vi "read_db_selected_events.vi"(8 "error in (no error)":errorcluster, 10 "Small?":bool, 11 "Dust Events":i64[](array[numeric])) -> (0 "error out":errorcluster, 1 "ID Experiment Settings":i32[](array[numeric]), 2 "ID Dust Events":i64[](array[numeric]), 3 "Dust Array":T2[](array[typedef]) {"File Location" items=["Unknown"=-1, "Processing"=0, "Storage"=1]; "Estimate Source" items=["Any Source."=-2, "No Shot"=-1, "Basic Labview Estimate"=0, "IDL Estimate From Andrew"=1, "IDL Estimate From Tobin"=2, "Old Metadata"=3]}, 5 "File Locations":T1[](array[typedef]) items=["Unknown"=-1, "Processing"=0, "Storage"=1])   [LabVIEW 2013]
doc: "Given a set of constraints, this program will return a lot of data about each event that matces the constraints."
uses:
  Public API/Query_Dust_Event.ctl
  Controls/Estimate_source.ctl
  Controls/File_location.ctl
  <userlib>/_OpenG.lib/array/array.llb/Empty 1D Array (I64)__ogtk.vi
  <userlib>/_OpenG.lib/array/array.llb/Reverse 2D Array (Variant)__ogtk.vi
  <vilib>/addons/database/_DB Variant To Data/Database Variant To Data.xnode
panel:
  out "SQL Query Syntax":string
  # "Dust Event"
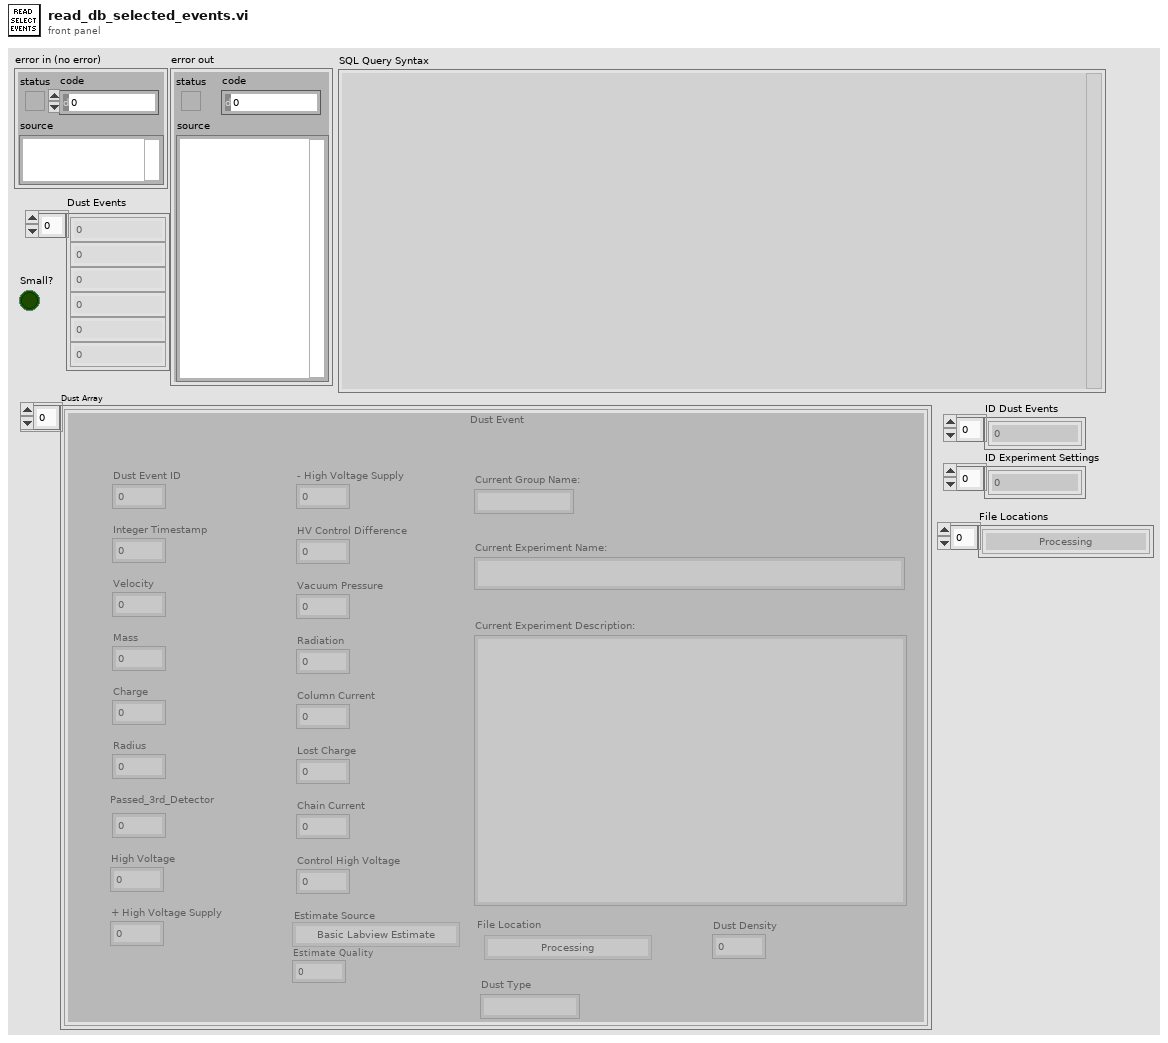
[diagram p1: front panel]
types:
  T1 = typedef "File_location.ctl" = i8
  T2 = typedef "Query_Dust_Event.ctl" = cluster{"Dust Event ID":i64, "Integer Timestamp":i64, "Velocity":sgl, "Mass":sgl, "Charge":sgl, "Radius":sgl, "Passed_3rd_Detector":i8, "High Voltage":sgl, "+ High Voltage Supply":sgl, "- High Voltage Supply":sgl, "HV Control Difference":sgl, "Vacuum Pressure":sgl, "Radiation":sgl, "Column Current":sgl, "Lost Charge":sgl, "Chain Current":sgl, "Control High Voltage":sgl, "Current Group Name:":string, "Current Experiment Name:":string, "Current Experiment Description:":string, "Estimate Source":T3, "Estimate Quality":i8, "File Location":T1, "Dust Type":string, "Dust Density":sgl}
  T3 = typedef "Estimate_source.ctl" = i8
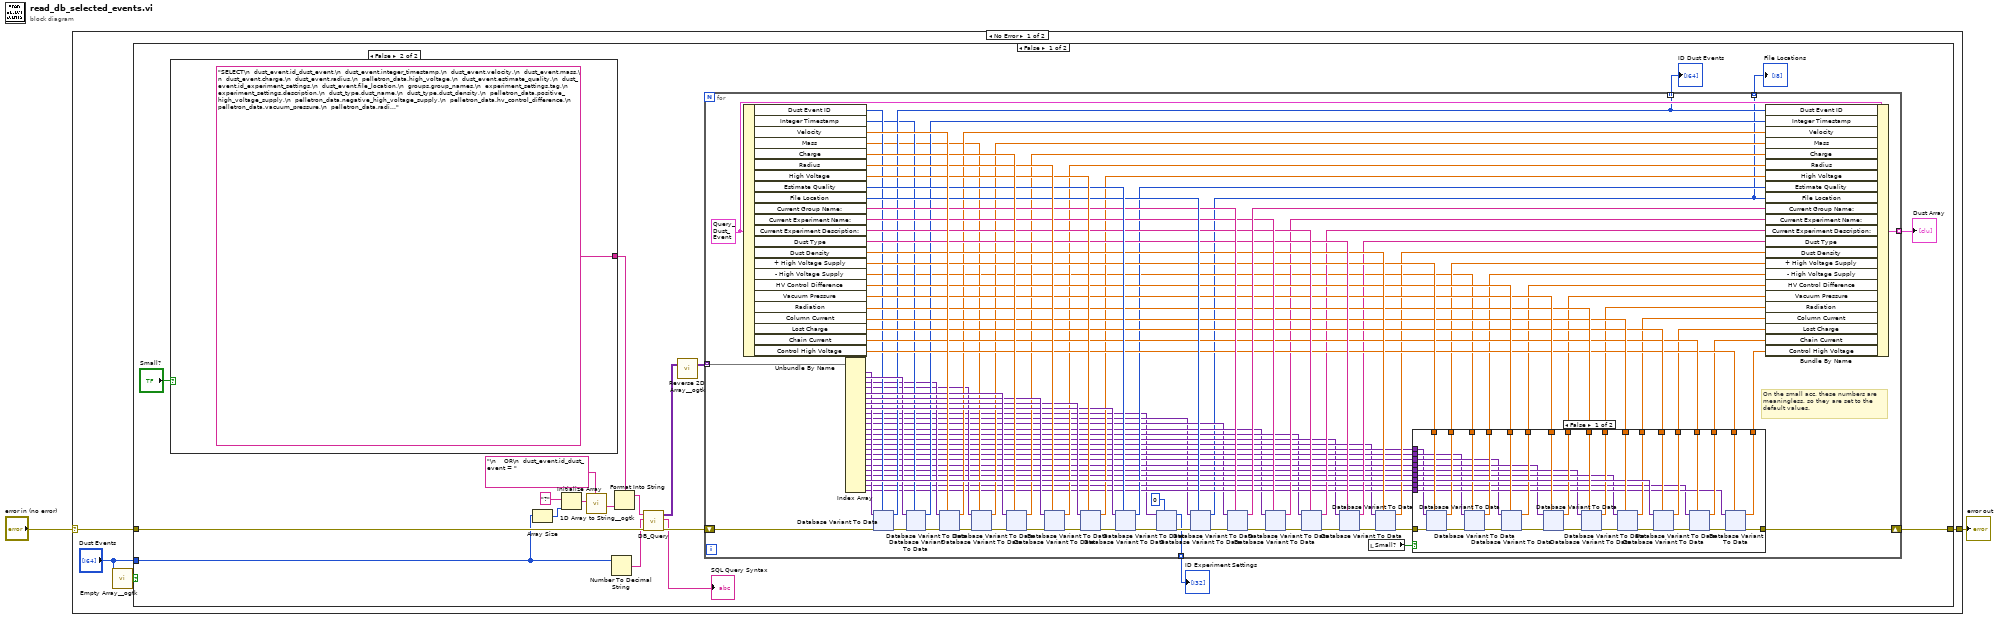
[diagram p0: block diagram]
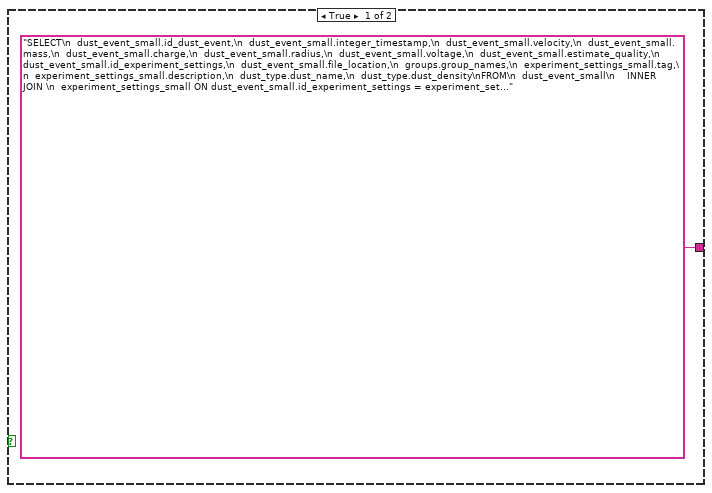
[diagram p3: hidden frame]
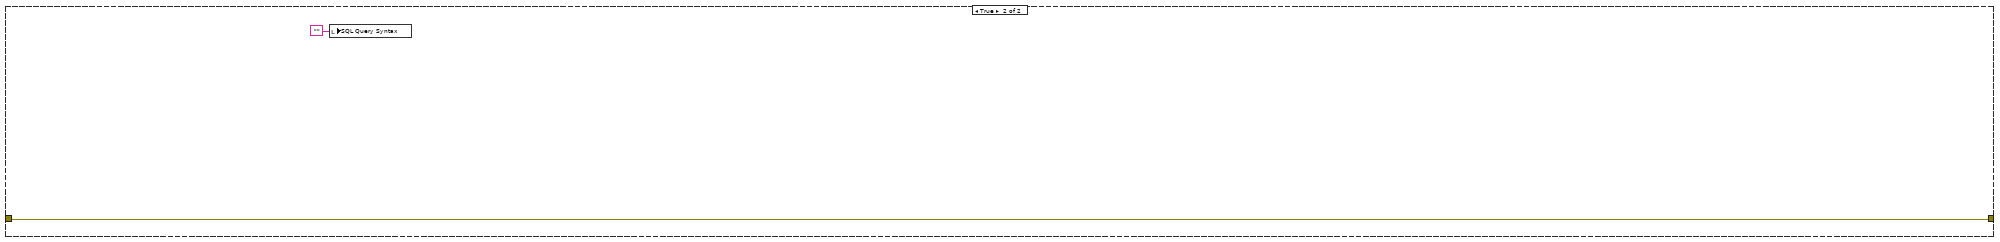
[diagram p4: hidden frame]
diagram:
  n1 = case shown="No Error" "error in (no error)" {
    selector: "error in (no error)" -> [w5 w939]
    tunnel: [w6 w939] -> w1
    frame No Error {
      n2 = call-poly <userlib>:"Empty Array__ogtk.vi"("Array"="Dust Events") -> ("Empty Array?"=w4:bool)  [unwired: 8 in]
      n3 = case shown="False" w4 {
        tunnel: [w24 w938] -> w6
        tunnel: w5 -> [w19 w938]
        tunnel: "Dust Events" -> [w17 _]
        frame False {
          n4 = case shown="False" "Small?" {
            tunnel: ["SELECT\n  dust_event_small.id_dust_event,\n  dust_event_small.integer_timestamp,\n  dust_event_small.velocity,\n  dust_event_small.mass,\n  dust_event_small.charge,\n  dust_event_small.radius,\n  dust_event_small.voltage,\n  dust_event_small.estimate_quality,\n  dust_event_small.id_experiment_settings,\n  dust_event_small.file_location,\n  groups.group_names,\n  experiment_settings_small.tag,\n  experiment_settings_small.description,\n  dust_type.dust_name,\n  dust_type.dust_density\nFROM\n  dust_event_small\n    INNER JOIN \n  experiment_settings_small ON dust_event_small.id_experiment_settings = experiment_settings_small.id_experiment_settings\n    INNER JOIN  \n  groups ON experiment_settings_small.id_groups=groups.id_groups\n    INNER JOIN\n  dust_info_small ON dust_event_small.id_dust_info = dust_info_small.id_dust_info\n  \t\tINNER JOIN\n  dust_type ON dust_info_small.dust_type = dust_type.id_dust_type\nWHERE\n  dust_event_small.id_dust_event = %s; " ("string") "SELECT\n  dust_event.id_dust_event,\n  dust_event.integer_timestamp,\n  dust_event.velocity,\n  dust_event.mass,\n  dust_event.charge,\n  dust_event.radius,\n  pelletron_data.high_voltage,\n  dust_event.estimate_quality,\n  dust_event.id_experiment_settings,\n  dust_event.file_location,\n  groups.group_names,\n  experiment_settings.tag,\n  experiment_settings.description,\n  dust_type.dust_name,\n  dust_type.dust_density,\n  pelletron_data.positive_high_voltage_supply,\n  pelletron_data.negative_high_voltage_supply,\n  pelletron_data.hv_control_difference,\n  pelletron_data.vacuum_pressure,\n  pelletron_data.radiation,\n  pelletron_data.column_current,\n  pelletron_data.lost_charge,\n  pelletron_data.chain_current,\n  pelletron_data.control_high_voltage\nFROM\n  dust_event\n    INNER JOIN \n  experiment_settings ON dust_event.id_experiment_settings = experiment_settings.id_experiment_settings\n    INNER JOIN  \n  groups ON experiment_settings.id_groups=groups.id_groups\n    INNER JOIN\n  pelletron_data ON pelletron_data.id_pelletron_data = dust_event.id_pelletron_data\n    INNER JOIN\n  dust_info ON dust_event.id_dust_info = dust_info.id_dust_info\n\t\t  INNER JOIN\n\t dust_type ON dust_info.dust_type = dust_type.id_dust_type\nWHERE\n  dust_event.id_dust_event = %s; " ("string")] -> w12
            frame True {
            }
            frame False {
            }
          }
          n5 = Array Size(array=w17) -> (size(s)=w15:i32)
          n6 = Initialize Array("?", w15) -> (w14:string[])
          n7 = call <userlib>:"1D Array to String__ogtk.vi"("delimiter (Tab)"="\n    OR\n  dust_event.id_dust_event = ", "Array of Strings"=w14) -> ("delimited string"=w10:string)  [unwired: 9 in]
          n8 = Number To Decimal String(number=w17) -> (decimal integer string=w18:string[])  [unwired: 1 in]
          n9 = Format Into String(format string=w12, w10) -> (resulting string=w11:string)  [unwired: 2 in, 1 out]
          n10 = call "DB_Query.vi"("error in (no error)"=w19, "Parameters"=w18, "Parameterized Query"=w11) -> ("error out"=w22:errorcluster, "Query in Standard Format"=→"SQL Query Syntax":string, "Results"=w21:variant[][])  [unwired: 6 in]
          n11 = call-poly <userlib>:"Reverse 2D Array__ogtk.vi"("Array"=w21) -> ("Reversed Array"=w23:variant[][])  [unwired: 2 in]
          n12 = for {
            tunnel: w23 -> [w119] mode=indexing
            shift-right: [w87] -> w24
            shift-left: w22 -> [w118]
            tunnel: [w92] -> w26 mode=indexing
            tunnel: [w79] -> w9 mode=indexing
            tunnel: [w29] -> w7 mode=indexing
            tunnel: [w28] -> w8 mode=indexing
            w117 = T2 {"Dust Event ID"=0, "Integer Timestamp"=0, "Velocity"=0.0, "Mass"=0.0, "Charge"=0.0, "Radius"=0.0, "Passed_3rd_Detector"=0, "High Voltage"=0.0, "+ High Voltage Supply"=0.0, "- High Voltage Supply"=0.0, "HV Control Difference"=0.0, "Vacuum Pressure"=0.0, "Radiation"=0.0, "Column Current"=0.0, "Lost Charge"=0.0, "Chain Current"=0.0, "Control High Voltage"=0.0, "Current Group Name:"="", "Current Experiment Name:"="", "Current Experiment Description:"="", "Estimate Source"=0, "Estimate Quality"=0, "File Location"=0, "Dust Type"="", "Dust Density"=0.0} ("Cluster")
            # "On the small acc, these numbers are\nmeaningless, so they are set to the\ndefault values."
            n13 = Unbundle By Name(w117) -> ("Dust Event ID"=w80:i64, "Integer Timestamp"=w78:i64, "Velocity"=w115:sgl, "Mass"=w73:sgl, "Charge"=w112:sgl, "Radius"=w108:sgl, "High Voltage"=w106:sgl, "Estimate Quality"=w104:i8, "File Location"=w103:T1, "Current Group Name:"=w102:string, "Current Experiment Name:"=w100:string, "Current Experiment Description:"=w99:string, "Dust Type"=w98:string, "Dust Density"=w97:sgl, "+ High Voltage Supply"=w96:sgl, "- High Voltage Supply"=w62:sgl, "HV Control Difference"=w95:sgl, "Vacuum Pressure"=w94:sgl, "Radiation"=w93:sgl, "Column Current"=w91:sgl, "Lost Charge"=w90:sgl, "Chain Current"=w89:sgl, "Control High Voltage"=w88:sgl)
            n14 = Index Array(array=w119) -> (element #1=w81:variant, element #2=w82:variant, element #3=w76:variant, element #4=w74:variant, element #5=w111:variant, element #6=w107:variant, element #7=w85:variant, element #8=w84:variant, element #9=w30:variant, element #10=w34:variant, element #11=w35:variant, element #12=w36:variant, element #13=w37:variant, element #14=w38:variant, element #15=w39:variant, element #16=w40:variant, element #17=w41:variant, element #18=w42:variant, element #19=w43:variant, element #20=w44:variant, element #21=w45:variant, element #22=w83:variant, element #23=w52:variant, element #24=w53:variant)  [unwired: 24 in]
            n15 = xnode "Database Variant To Data"("database variant"=w81, "error in (no error)"=w118, "type"=w80) -> ("data"=w79:i64, "error out"=w116:errorcluster)
            n16 = xnode "Database Variant To Data"("database variant"=w82, "error in (no error)"=w116, "type"=w78) -> ("data"=w77:i64, "error out"=w114:errorcluster)
            n17 = xnode "Database Variant To Data"("database variant"=w76, "error in (no error)"=w114, "type"=w115) -> ("data"=w75:sgl, "error out"=w113:errorcluster)
            n18 = xnode "Database Variant To Data"("database variant"=w74, "error in (no error)"=w113, "type"=w73) -> ("data"=w72:sgl, "error out"=w110:errorcluster)
            n19 = xnode "Database Variant To Data"("database variant"=w111, "error in (no error)"=w110, "type"=w112) -> ("data"=w71:sgl, "error out"=w109:errorcluster)
            n20 = xnode "Database Variant To Data"("database variant"=w107, "error in (no error)"=w109, "type"=w108) -> ("data"=w70:sgl, "error out"=w86:errorcluster)
            n21 = xnode "Database Variant To Data"("database variant"=w85, "error in (no error)"=w86, "type"=w106) -> ("data"=w69:sgl, "error out"=w105:errorcluster)
            n22 = xnode "Database Variant To Data"("database variant"=w84, "error in (no error)"=w105, "type"=w104) -> ("data"=w68:i8, "error out"=w32:errorcluster)
            n23 = xnode "Database Variant To Data"("database variant"=w30, "error in (no error)"=w32, "type"=0 ("data")) -> ("data"=w29:i32, "error out"=w33:errorcluster)
            n24 = xnode "Database Variant To Data"("database variant"=w34, "error in (no error)"=w33, "type"=w103) -> ("data"=w28:T1, "error out"=w51:errorcluster)
            n25 = xnode "Database Variant To Data"("database variant"=w35, "error in (no error)"=w51, "type"=w102) -> ("data"=w101:string, "error out"=w50:errorcluster)
            n26 = xnode "Database Variant To Data"("database variant"=w36, "error in (no error)"=w50, "type"=w100) -> ("data"=w67:string, "error out"=w49:errorcluster)
            n27 = xnode "Database Variant To Data"("database variant"=w37, "error in (no error)"=w49, "type"=w99) -> ("data"=w66:string, "error out"=w48:errorcluster)
            n28 = xnode "Database Variant To Data"("database variant"=w38, "error in (no error)"=w48, "type"=w98) -> ("data"=w65:string, "error out"=w47:errorcluster)
            n29 = local read "Small?"() -> (w27:bool)
            n30 = xnode "Database Variant To Data"("database variant"=w39, "error in (no error)"=w47, "type"=w97) -> ("data"=w64:sgl, "error out"=w46:errorcluster)
            n31 = case shown="False" w27 {
              tunnel: w96 -> [w156 w454]
              tunnel: w95 -> [w154 w452]
              tunnel: w94 -> [w152 w451]
              tunnel: w93 -> [w151 w450]
              tunnel: w91 -> [w150 w449]
              tunnel: w90 -> [w149 w448]
              tunnel: w89 -> [w147 w447]
              tunnel: w88 -> [w146 w446]
              tunnel: [w144 w445] -> w87
              tunnel: w83 -> [w141 _]
              tunnel: [w140 w454] -> w63
              tunnel: w62 -> [w139 w453]
              tunnel: [w138 w453] -> w61
              tunnel: [w137 w452] -> w60
              tunnel: [w136 w451] -> w59
              tunnel: [w135 w450] -> w58
              tunnel: [w134 w449] -> w57
              tunnel: [w133 w448] -> w56
              tunnel: [w132 w447] -> w55
              tunnel: [w131 w446] -> w54
              tunnel: w53 -> [w130 _]
              tunnel: w52 -> [w129 _]
              tunnel: w46 -> [w128 w445]
              tunnel: w45 -> [w125 _]
              tunnel: w44 -> [w124 _]
              tunnel: w43 -> [w123 _]
              tunnel: w42 -> [w122 _]
              tunnel: w41 -> [w121 _]
              tunnel: w40 -> [w120 _]
              frame False {
                n32 = xnode "Database Variant To Data"("database variant"=w120, "error in (no error)"=w128, "type"=w156) -> ("data"=w140:sgl, "error out"=w127:errorcluster)
                n33 = xnode "Database Variant To Data"("database variant"=w121, "error in (no error)"=w127, "type"=w139) -> ("data"=w138:sgl, "error out"=w155:errorcluster)
                n34 = xnode "Database Variant To Data"("database variant"=w122, "error in (no error)"=w155, "type"=w154) -> ("data"=w137:sgl, "error out"=w153:errorcluster)
                n35 = xnode "Database Variant To Data"("database variant"=w123, "error in (no error)"=w153, "type"=w152) -> ("data"=w136:sgl, "error out"=w142:errorcluster)
                n36 = xnode "Database Variant To Data"("database variant"=w124, "error in (no error)"=w142, "type"=w151) -> ("data"=w135:sgl, "error out"=w143:errorcluster)
                n37 = xnode "Database Variant To Data"("database variant"=w125, "error in (no error)"=w143, "type"=w150) -> ("data"=w134:sgl, "error out"=w126:errorcluster)
                n38 = xnode "Database Variant To Data"("database variant"=w141, "error in (no error)"=w126, "type"=w149) -> ("data"=w133:sgl, "error out"=w145:errorcluster)
                n39 = xnode "Database Variant To Data"("database variant"=w129, "error in (no error)"=w145, "type"=w147) -> ("data"=w132:sgl, "error out"=w148:errorcluster)
                n40 = xnode "Database Variant To Data"("database variant"=w130, "error in (no error)"=w148, "type"=w146) -> ("data"=w131:sgl, "error out"=w144:errorcluster)
              }
              frame True {
              }
            }
            n41 = Bundle By Name(cluster=w117, "Dust Event ID"=w79, "Integer Timestamp"=w77, "Velocity"=w75, "Mass"=w72, "Charge"=w71, "Radius"=w70, "High Voltage"=w69, "Estimate Quality"=w68, "File Location"=w28, "Current Group Name:"=w101, "Current Experiment Name:"=w67, "Current Experiment Description:"=w66, "Dust Type"=w65, "Dust Density"=w64, "+ High Voltage Supply"=w63, "- High Voltage Supply"=w61, "HV Control Difference"=w60, "Vacuum Pressure"=w59, "Radiation"=w58, "Column Current"=w57, "Lost Charge"=w56, "Chain Current"=w55, "Control High Voltage"=w54) -> (w92:T2)
          }
          "Dust Array" <- w26
          "ID Dust Events" <- w9
          "File Locations" <- w8
          "ID Experiment Settings" <- w7
        }
        frame True {
          n42 = local write "SQL Query Syntax"("") -> ()
        }
      }
    }
    frame Error {
    }
  }
  "error out" <- w1
